vi "LJM logger append cfg if not exist.vi"(1 "Input String":string) -> (0 "Output String":string)   [LabVIEW 2026]
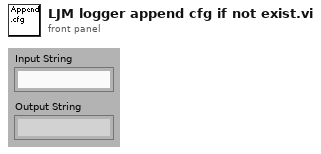
[diagram p1: front panel]
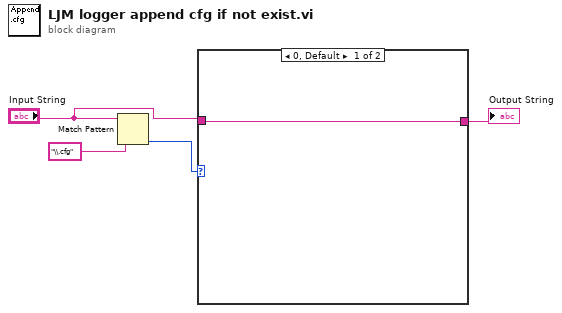
[diagram p0: block diagram]
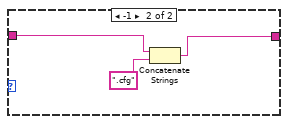
[diagram p2: hidden frame]
diagram:
  n1 = Match Pattern(string="Input String", regular expression="\\.cfg") -> (offset past match=w3:i32)  [unwired: 1 in, 3 out]
  n2 = case shown="0, Default" w3 {
    tunnel: "Input String" -> [w5 w7]
    tunnel: [w5 w6] -> w1
    frame 0, Default {
    }
    frame -1 {
      n3 = Concatenate Strings(w7, ".cfg" ("string")) -> (w6:string)
    }
  }
  "Output String" <- w1
